vi "breakBeam.vi"(6 "Falling Edge":bool, 7 "Rising Edge":bool, 8 "Distance between sensors(in)":dbl, 10 "BreakBeam2":T1, 11 "BreakBeam1":T1) -> (3 "Speed (distance/time) (ft/sec)":dbl)   [LabVIEW 2011]
uses:
  <vilib>/Rock Robotics/WPI/DigitalInput/WPI_DigitalInputDevRef.ctl
  <vilib>/Rock Robotics/SystemInterfaces/DIO/FPGA_DIOChannel.ctl
  <vilib>/Rock Robotics/SystemInterfaces/Typedef/FPGA_TypedefDigitalModule.ctl
  <vilib>/Rock Robotics/WPI/Counter/WPI_CounterDigitalInputToDigitalSource.vi
  Robot Global Data.vi
panel:
  out "Beam 2":bool
  out "Beam 1":bool
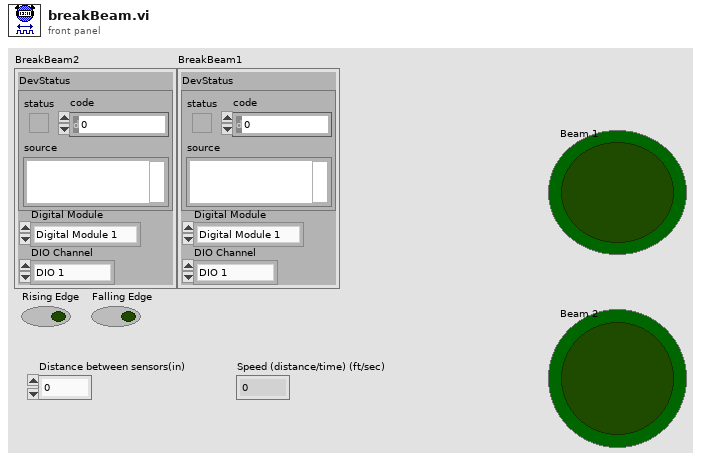
[diagram p1: front panel]
types:
  T1 = typedef "WPI_DigitalInputDevRef.ctl" = cluster{"DevStatus":errorcluster, "DIO Channel":T2, "Digital Module":T3}
  T2 = typedef "FPGA_DIOChannel.ctl" = enum8{"DIO 1", "DIO 2", "DIO 3", "DIO 4", "DIO 5", "DIO 6", "DIO 7", "DIO 8", "DIO 9", "DIO 10", "DIO 11", "DIO 12", "DIO 13", "DIO 14", "Invalid"}
  T3 = typedef "FPGA_TypedefDigitalModule.ctl" = enum16{"Digital Module 1", "Digital Module 2"}
  T4 = typedef "FPGA_CounterEncoderSourceConvertionLVSourceType.ctl" = cluster{"DevStatus":errorcluster, "AnalogTriggerMode?":bool, "DigitalMode":cluster{"Digital Module":T3, "DIO Channel":T5}, "AnalogTriggerMode":cluster{"AnalogTriggerIndex":T6, "OutputType":T7}}
  T5 = typedef "FPGA_DIODigitalSourceChannel.ctl" = enum8{"DIO 1", "DIO 2", "DIO 3", "DIO 4", "DIO 5", "DIO 6", "DIO 7", "DIO 8", "DIO 9", "DIO 10", "DIO 11", "DIO 12", "DIO 13", "DIO 14", "Disabled"}
  T6 = typedef "FPGA_AnalogTriggerIndex.ctl" = enum8{"Trig 0", "Trig 1", "Trig 2", "Trig 3", "Trig 4", "Trig 5", "Trig 6", "Trig 7", "Invalid"}
  T7 = typedef "FPGA_AnalogTriggerOutType.ctl" = enum16{"InWindow", "TriggerState", "Rising", "Falling"}
  T8 = typedef "WPI_InterruptRef.ctl" = cluster{"DevStatus":errorcluster, "InterruptIndex":T9}
  T9 = typedef "FPGA_InterruptIndex.ctl" = enum8{"0", "1", "2", "3", "4", "5", "6", "7", "Invalid"}
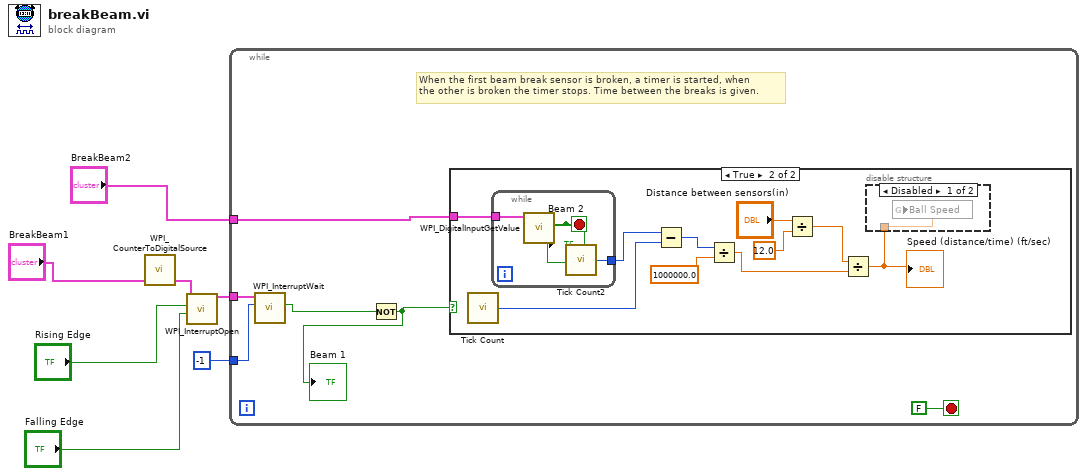
[diagram p0: block diagram]
diagram:
  n1 = call-poly <vilib>:"WPI_CounterToDigitalSource.vi"("DigitalInputDevRef"="BreakBeam1") -> ("Digital Source"=w7:T4)  [unwired: 6 in]
  n2 = call <vilib>:"WPI_InterruptOpen.vi"("Falling Edge"="Falling Edge", "Rising Edge"="Rising Edge", "Source"=w7) -> ("InterruptRef"=w6:T8)  [unwired: 7 in, 1 out]
  n3 = while {
    tunnel: "BreakBeam2" -> [w13]
    tunnel: w6 -> [w11]
    tunnel: -1 ("Timeout (ms)") -> [w10]
    stop <- FALSE stop-if-true
    # "When the first beam break sensor is broken, a timer is started, when\nthe other is broken the timer stops. Time between the breaks is given."
    n4 = call <vilib>:"WPI_InterruptWait.vi"("Timeout (ms)"=w10, "InterruptRef"=w11) -> ("Timed Out"=w12:bool)  [unwired: 6 in, 3 out]
    n5 = Not(x=w12) -> (.not. x?=w8:bool)
    "Beam 1" <- w8
    n6 = case shown="True" w8 {
      tunnel: w13 -> [_ w23]
      frame False {
      }
      frame True {
        n7 = call "Tick Count"() -> ("Tick Count(uSec)"=w19:u32)
        n8 = while {
          tunnel: w23 -> [w27]
          tunnel: [w25] -> w20
          stop <- w26 stop-if-true
          n9 = call <vilib>:"WPI_DigitalInputGetValue.vi"("DigitalInputDevRef"=w27) -> ("Value"=w26:bool)  [unwired: 8 in, 2 out]
          "Beam 2" <- w26
          n10 = call "Tick Count2"() -> ("Tick Count(uSec)"=w25:u32)
        }
        n11 = Subtract(x=w20, y=w19) -> (x-y=w21:u32)
        n12 = Divide(x=w21, y=1000000.0) -> (x/y=w18:dbl)
        n13 = Divide(x="Distance between sensors(in)", y=12.0) -> (x/y=w15:dbl)
        n14 = Divide(x=w15, y=w18) -> (x/y=w14:dbl)
        "Speed (distance/time) (ft/sec)" <- w14
        n15 = disable-structure shown="Disabled" {
          disable-tunnel: w14 -> [w24 _]
          frame Disabled {
            n16 = global write "Robot Global Data.vi" "Ball Speed"(w24) -> ()
          }
          frame Enabled {
          }
        }
      }
    }
  }
